vi "test.vi"() -> ()   [LabVIEW 2009]
panel:
  out "appended array":dbl[][](array[numeric])
  out "Data HFWM":dbl[][](array[numeric])
  out "Temperature":dbl[][](array[numeric])
  out "Secondary Delay":dbl[](array[numeric])
  out "Primary Delay":dbl[](array[numeric])
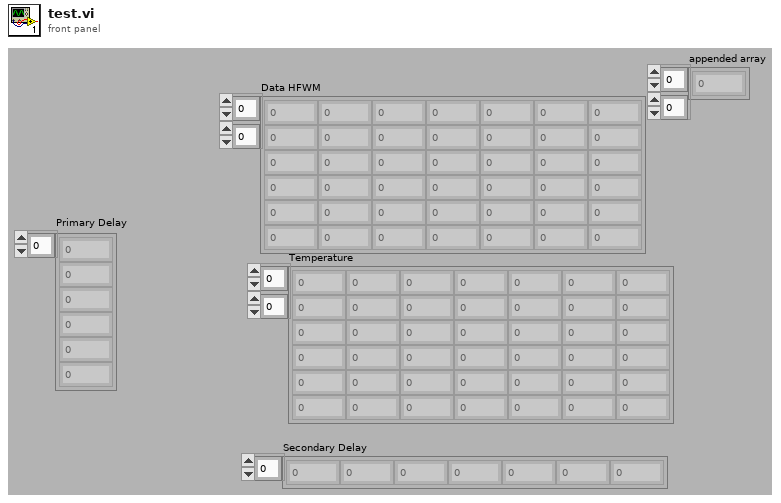
[diagram p1: front panel]
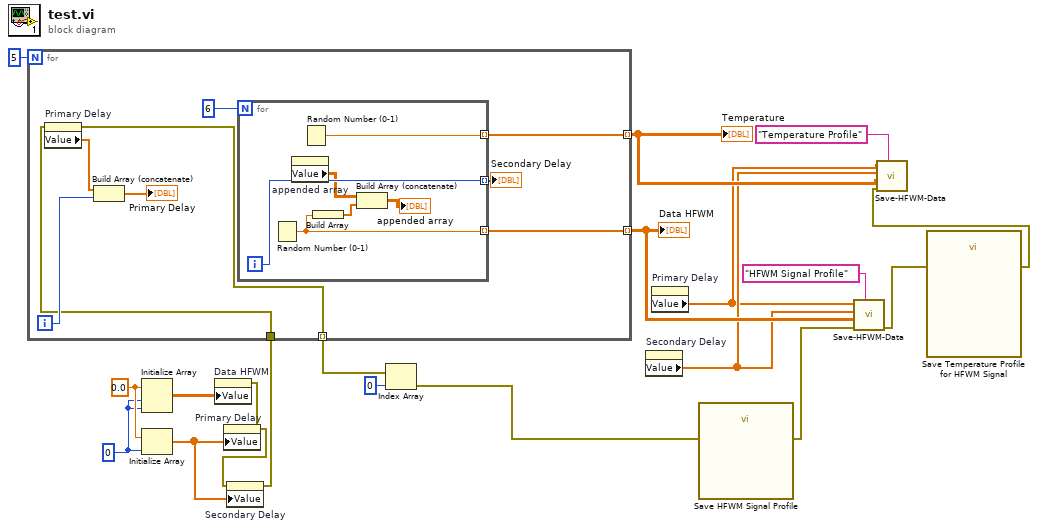
[diagram p0: block diagram]
diagram:
  w18 = 0 ("dimension size")
  w19 = 0.0 ("element")
  n1 = Initialize Array(w19, w18, w18) -> (w16:dbl[][])
  n2 = Initialize Array(w19, w18) -> (w17:dbl[])
  n3 = property on="Data HFWM" class="Arr (strict)"("Value"=w16) -> (error out=w15:errorcluster)  [unwired: 2 in, 1 out]
  n4 = property on="Primary Delay" class="Arr (strict)"(error in=w15, "Value"=w17) -> (error out=w14:errorcluster)  [unwired: 1 in, 1 out]
  n5 = property on="Secondary Delay" class="Arr (strict)"(error in=w14, "Value"=w17) -> (error out=w4:errorcluster)  [unwired: 1 in, 1 out]
  n6 = for {
    N: 5 -> [_]
    tunnel: [w23] -> w11 mode=indexing
    tunnel: [w25] -> w13 mode=indexing
    tunnel: w4 -> [w24]
    tunnel: [w21] -> w3 mode=indexing
    i -> [w26]
    n7 = property on="Primary Delay" class="Arr (strict)"(error in=w24) -> (error out=w21:errorcluster, "Value"=w27:dbl[])  [unwired: 1 in, 1 out]
    n8 = Build Array (concatenate)(w27, w26) -> (→"Primary Delay":dbl[])
    n9 = for {
      N: 6 -> [_]
      tunnel: [w34] -> w22 mode=indexing
      tunnel: [w35] -> w23 mode=indexing
      tunnel: [w33] -> w25 mode=indexing
      i -> [w34]
      n10 = Random Number (0-1)() -> (number: 0 to 1=w33:dbl)
      n11 = property on="appended array" class="Arr (strict)"() -> ("Value"=w30:dbl[][])  [unwired: 2 in, 2 out]
      n12 = Random Number (0-1)() -> (number: 0 to 1=w35:dbl)
      n13 = Build Array(w33) -> (w32:dbl[])
      n14 = Build Array (concatenate)(w30, w32) -> (→"appended array":dbl[][])
    }
    "Secondary Delay" <- w22
  }
  "Temperature" <- w11
  "Data HFWM" <- w13
  n15 = Index Array(array=w3, index=0) -> (element=w1:errorcluster)
  n16 = property on="Secondary Delay" class="Arr (strict)"() -> ("Value"=w10:dbl[])  [unwired: 2 in, 2 out]
  n17 = property on="Primary Delay" class="Arr (strict)"() -> ("Value"=w9:dbl[])  [unwired: 2 in, 2 out]
  n18 = call "Save HFWM Signal Profile"("error in (no error)"=w1) -> ("error out"=w5:errorcluster)  [unwired: 17 in, 1 out]
  n19 = call "Save-HFWM-Data.vi"("Data Profile Name"="HFWM Signal Profile", "error in (no error)"=w5, "Data:"=w13, "Secondary Delay"=w10, "Primary Delay"=w9) -> ("error out"=w6:errorcluster)  [unwired: 6 in]
  n20 = call "Save Temperature Profile for HFWM Signal"("error in (no error)"=w6) -> ("error out"=w12:errorcluster)  [unwired: 17 in, 1 out]
  n21 = call "Save-HFWM-Data.vi"("Data Profile Name"="Temperature Profile", "error in (no error)"=w12, "Data:"=w11, "Secondary Delay"=w10, "Primary Delay"=w9) -> ()  [unwired: 6 in, 1 out]
